vi "Shorting of Test Seq Program.vi"(5 "Feature List (Out)":T1(array[cluster])) -> (1 "Feature Step Enable":T1(array[cluster]), 2 "Feature Name":string[][](array[string]))   [LabVIEW 2015]
panel:
  out "Pokayoka Result":cluster{"Sensor Name":string, "Boolean":bool}[](array[cluster])
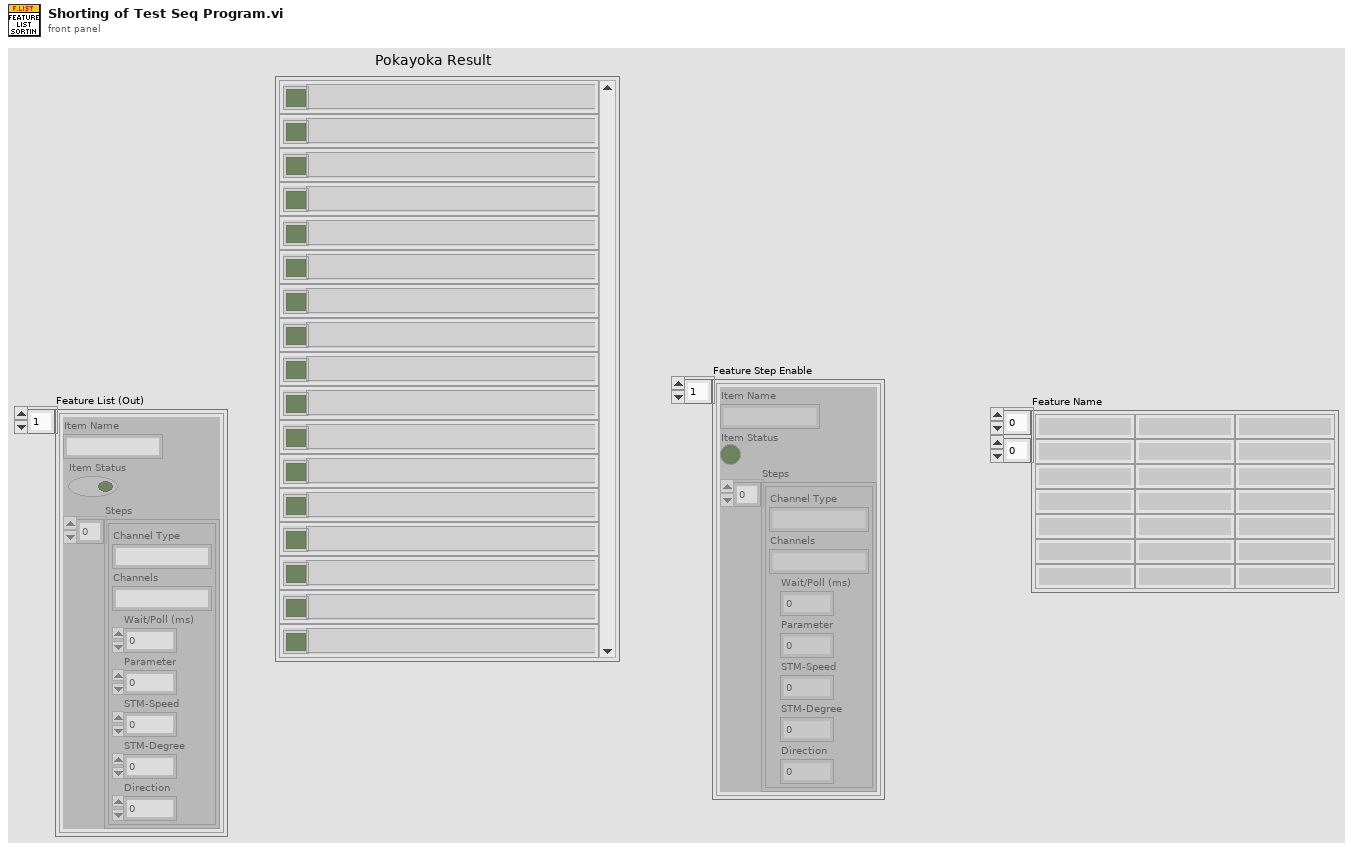
[diagram p1: front panel]
types:
  T1 = cluster{"Item Name":string, "Item Status":bool, "Steps":cluster{"Channel Type":string, "Channels":string, "Wait/Poll (ms)":u32, "Parameter":u8, "STM-Speed":i32, "STM-Degree":u32, "Direction":u8}[]}[]
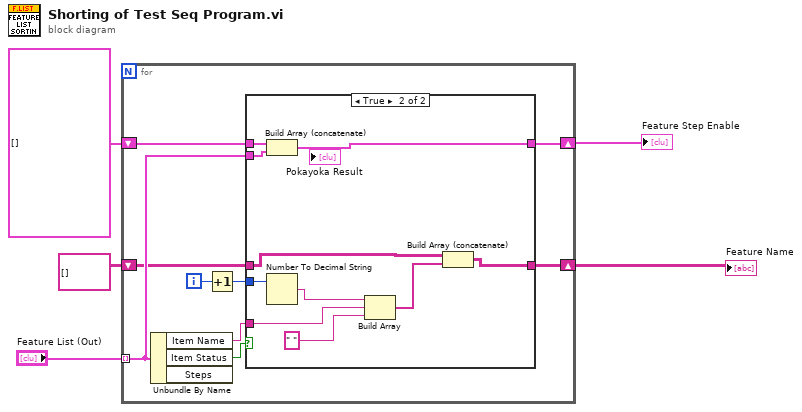
[diagram p0: block diagram]
diagram:
  n1 = for {
    tunnel: "Feature List (Out)" -> [w12] mode=indexing
    shift-right: [w9] -> w1
    shift-left: string[][] [] -> [w8]
    shift-right: [w7] -> w3
    shift-left: T1 [] -> [w6]
    i -> [w11]
    n2 = Unbundle By Name(w12) -> ("Item Name"=w13:string, "Item Status"=w14:bool)  [unwired: 1 out]
    n3 = Increment(x=w11) -> (x+1=w10:i32)
    n4 = case shown="True" w14 {
      tunnel: w13 -> [_ w26]
      tunnel: w12 -> [_ w22]
      tunnel: w10 -> [_ w25]
      tunnel: [w16 w24] -> w9
      tunnel: w8 -> [w16 w23]
      tunnel: [w15 w21] -> w7
      tunnel: w6 -> [w15 w20]
      frame False {
      }
      frame True {
        n5 = Build Array (concatenate)(w20, w22) -> (w21:T1)
        n6 = Number To Decimal String(number=w25) -> (decimal integer string=w19:string)  [unwired: 1 in]
        n7 = Build Array(w19, w26, " " ("element")) -> (w17:string[])
        n8 = Build Array (concatenate)(w23, w17) -> (w24:string[][])
      }
    }
  }
  "Feature Name" <- w1
  "Feature Step Enable" <- w3
